vi "InitIMU.vi"(8 "error in (no error)":errorcluster) -> (0 "error out":errorcluster, 2 "Acc/Gyro  address":u8, 3 "I2C Ref Out":T1)   [LabVIEW 2019]
uses:
  <vilib>/myRIO/Instrument Drivers/Onboard IO/I2C/typedefs/I2C Reference.ctl
  <vilib>/myRIO/Common/Instrument Driver Framework/Utilities/typedefs/myRIO Generic Hardware Reference.ctl
  <vilib>/myRIO/Common/Instrument Driver Framework/Utilities/typedefs/Hardware Version Enum.ctl
  <vilib>/myRIO/Common/Instrument Driver Framework/Utilities/typedefs/myRIO v1.0 Reference.ctl
  <vilib>/myRIO/Common/Instrument Driver Framework/Utilities/typedefs/Generic FPGA Reference.ctl
  <vilib>/myRIO/Common/Instrument Driver Framework/myRIO v1.0/I2C/typedefs/I2C Channels Enum.ctl
  <vilib>/myRIO/Instrument Drivers/Onboard IO/I2C/typedefs/I2C Configuration.ctl
  <vilib>/myRIO/Instrument Drivers/Onboard IO/I2C/typedefs/I2C Transfer Rate.ctl
  <vilib>/myRIO/Instrument Drivers/Onboard IO/I2C/typedefs/I2C User Configuration.ctl
  <vilib>/Utility/error.llb/Error Cluster From Error Code.vi
  <vilib>/myRIO/Common/Instrument Driver Framework/myRIO v1.0/I2C/vis/myRIO v1.0 Configure I2C.vi
  <vilib>/myRIO/Common/Instrument Driver Framework/myRIO v1.0/I2C/vis/myRIO v1.0 Write I2C.vi
  <vilib>/myRIO/Instrument Drivers/Onboard IO/I2C/I2C.lvlib
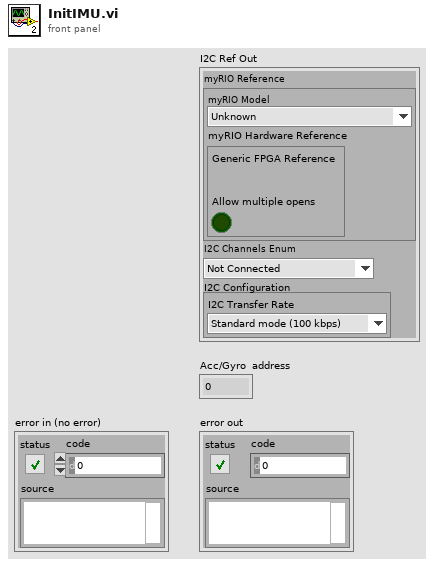
[diagram p1: front panel]
types:
  T1 = typedef "I2C.lvlib/I2C Reference.ctl" = cluster{"myRIO Reference":T2, "I2C Channels Enum":T6, "I2C Configuration":T7}
  T2 = typedef "myRIO Generic Hardware Reference.ctl" = cluster{"myRIO Model":T3, "myRIO Hardware Reference":T4}
  T3 = typedef "Hardware Version Enum.ctl" = enum16{"Unknown", "myRIO-1900", "myRIO-1950", "roboRIO", "NI ELVIS RIO CM", "ELVIS III"}
  T4 = typedef "myRIO v1.0 Reference.ctl" = cluster{"Generic FPGA Reference":T5, "Allow multiple opens":bool}
  T5 = typedef "Generic FPGA Reference.ctl" = refnum<k20>
  T6 = typedef "I2C Channels Enum.ctl" = enum16{"Not Connected", "A/I2C", "B/I2C", "I2C/I2C"}
  T7 = typedef "I2C.lvlib/I2C Configuration.ctl" = cluster{"I2C Transfer Rate":T8}
  T8 = typedef "I2C.lvlib/I2C Transfer Rate.ctl" = enum16{"Standard mode (100 kbps)", "Fast mode (400 kbps)"}
  T9 = typedef "I2C.lvlib/I2C User Configuration.ctl" = cluster{"I2C Transfer Rate":T8}
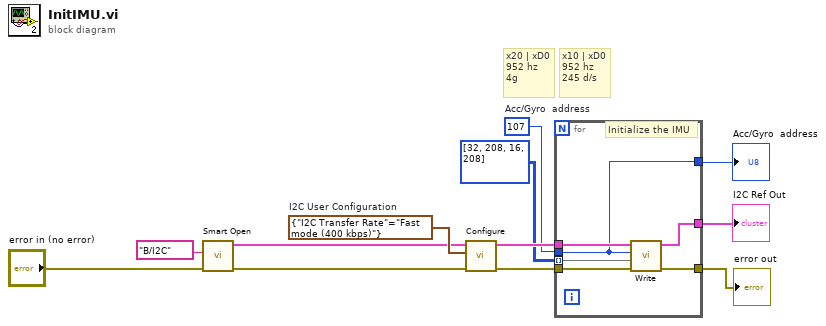
[diagram p0: block diagram]
diagram:
  w4 = u8 107  # Acc/Gyro  address
  w12 = T9 {"I2C Transfer Rate"=enum."Fast mode (400 kbps)"}  # I2C User Configuration
  # "x20 | xD0\n952 hz\n4g"
  # "x10 | xD0\n952 hz\n245 d/s"
  n1 = call <vilib>:"Smart Open.vi"("error in (no error)"="error in (no error)", "Channel Name"=tag "B/I2C" ("I2C I/O")) -> ("error out"=w1:errorcluster, "I2C Ref Out"=w2:T1)  [unwired: 8 in]
  n2 = call <vilib>:"Configure.vi"("error in (no error)"=w1, "I2C User Configuration"=w12, "I2C Ref In"=w2) -> ("error out"=w10:errorcluster, "I2C Ref Out"=w11:T1)  [unwired: 7 in]
  n3 = for {
    tunnel: [w17] -> w8
    tunnel: [w18] -> w7
    tunnel: u8[][] [[32, 208], [16, 208]] ("Bytes to Write") -> [w16] mode=indexing
    tunnel: w4 -> [w13]
    tunnel: w11 -> [w15]
    tunnel: w10 -> [w14]
    tunnel: [w13] -> w6
    # "Initialize the IMU"
    n4 = call <vilib>:"Write.vi"("error in (no error)"=w14, "Bytes to Write"=w16, "Slave Address (7-bit)"=w13, "I2C Ref In"=w15) -> ("error out"=w17:errorcluster, "I2C Ref Out"=w18:T1)  [unwired: 6 in]
  }
  "error out" <- w8
  "I2C Ref Out" <- w7
  "Acc/Gyro  address" <- w6
